vi "Display Charm.vi"(8 "error in (no error)":errorcluster, 9 "Charm Enqueuer":refnum<class "Message Enqueuer.lvclass">, 11 "MainController in":refnum<class "MainController.lvclass">) -> (0 "error out":errorcluster, 3 "MainController out":refnum<class "MainController.lvclass">)   [LabVIEW 2012, in "Win8uiFramework.lvlib" / "MainController.lvclass"]
uses:
  MainController.lvclass
  <vilib>/ActorFramework/Message Enqueuer/Message Enqueuer.lvclass
  Visibility Direction.ctl
  Visiblity States.ctl
  MainController.lvclass/MainController.ctl
  Insert Into SubPanel Msg.lvclass/Insert Into SubPanel Msg.ctl
  <vilib>/ActorFramework/Message Enqueuer/Message Enqueuer.lvclass/Message Enqueuer.ctl
  Read Charm SubPanel.vi
  Read Charm Enqueuer.vi
  Read Charm State.vi
  Write Charm Enqueuer.vi
  Write Charm State.vi
  <vilib>/ActorFramework/Message Enqueuer/Enqueue.vi
  <vilib>/ActorFramework/Message Priority Queue/Priority Enqueue.vi
  <vilib>/Utility/error.llb/Simple Error Handler.vi
  Insert Into SubPanel Msg.lvclass
  Win8uiFramework.lvlib
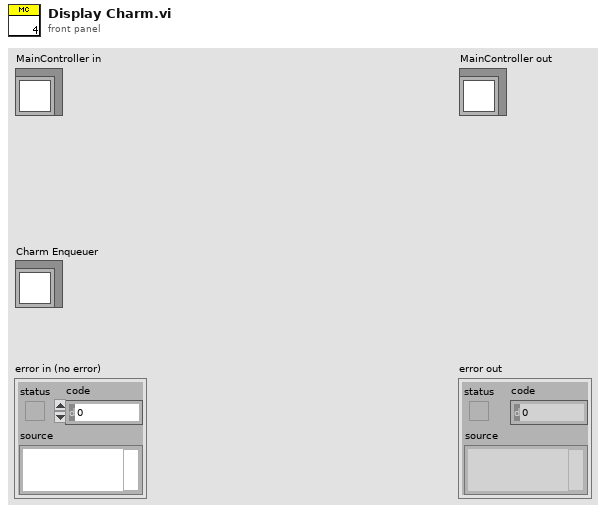
[diagram p1: front panel]
types:
  T1 = typedef "Win8uiFramework.lvlib/MainController.lvclass/Visiblity States.ctl" = enum16{"Disabled", "Hidden - Unpopulated", "Hidden - Populated", "Visible"}
  T2 = typedef "Win8uiFramework.lvlib/Visibility Direction.ctl" = enum16{"Show", "Hide"}
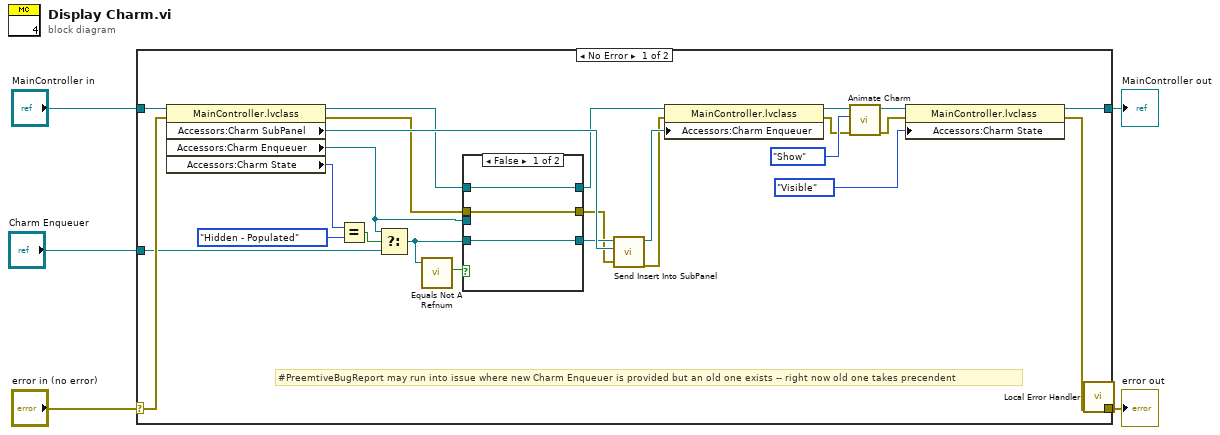
[diagram p0: block diagram]
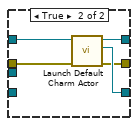
[diagram p2: hidden frame]
diagram:
  n1 = case shown="No Error" "error in (no error)" {
    selector: "error in (no error)" -> [w28 w41]
    tunnel: [w8 w41] -> w4
    tunnel: [w22 w40] -> w2
    tunnel: "MainController in" -> [w31 w40]
    tunnel: "Charm Enqueuer" -> [w19 _]
    frame No Error {
      # "#PreemtiveBugReport may run into issue where new Charm Enqueuer is provided but an old one exists -- right now old one takes precendent"
      n2 = property class="MainController.lvclass"(reference=w31, error in=w28) -> (reference out=w11:refnum<class "MainController.lvclass">, error out=w13:errorcluster, "Accessors:Charm SubPanel"=w30:refnum<vi>, "Accessors:Charm Enqueuer"=w6:refnum<class "Message Enqueuer.lvclass">, "Accessors:Charm State"=w18:T1)
      n3 = Equal?(x=w18, y=Visiblity_States."Hidden - Populated") -> (x = y?=w7:bool)
      n4 = Select(t=w6, s=w7, f=w19) -> (s? t:f=w16:refnum<class "Message Enqueuer.lvclass">)
      n5 = call <vilib>:"Equals Not A Refnum.vi"("Message Enqueuer"=w16) -> ("Not a refnum?"=w14:bool)  [unwired: 10 in]
      n6 = case shown="False" w14 {
        tunnel: w16 -> [w34 _]
        tunnel: [w34 w39] -> w15
        tunnel: w11 -> [w32 w37]
        tunnel: w13 -> [w33 w38]
        tunnel: [w32 w36] -> w10
        tunnel: [w33 w35] -> w12
        tunnel: w6 -> [_ _]
        frame False {
        }
        frame True {
          n7 = call-dynamic "Launch Default Charm Actor.vi"("error in (no error)"=w38, "MainController in"=w37) -> ("error out"=w35:errorcluster, "Enqueuer"=w39:refnum<class "Message Enqueuer.lvclass">, "MainController out"=w36:refnum<class "MainController.lvclass">)  [unwired: 7 in]
        }
      }
      n8 = call "Send Insert Into SubPanel.vi"("error in (no error)"=w12, "SubPanel Ref"=w30, "Message Enqueuer"=w15) -> ("error out"=w27:errorcluster, "Message Enqueuer out"=w29:refnum<class "Message Enqueuer.lvclass">)  [unwired: 7 in]
      n9 = property class="MainController.lvclass"(reference=w10, error in=w27, "Accessors:Charm Enqueuer"=w29) -> (reference out=w26:refnum<class "MainController.lvclass">, error out=w24:errorcluster)
      n10 = call-dynamic "Animate Charm.vi"("error in (no error)"=w24, "Direction"=Visibility_Direction."Show", "MainController in"=w26) -> ("error out"=w20:errorcluster, "MainController out"=w23:refnum<class "MainController.lvclass">)  [unwired: 7 in]
      n11 = property class="MainController.lvclass"(reference=w23, error in=w20, "Accessors:Charm State"=Visiblity_States."Visible" ("Charm State")) -> (reference out=w22:refnum<class "MainController.lvclass">, error out=w9:errorcluster)
      n12 = call "Local Error Handler.vi"("error in (no error)"=w9) -> ("error out"=w8:errorcluster)  [unwired: 18 in]
    }
    frame Error {
    }
  }
  "error out" <- w4
  "MainController out" <- w2
